vi "VertRead_import_SM1_full_control_100step_camtrigger.vi"() -> ()   [LabVIEW 2021]
uses:
  <vilib>/DAQmx/write.llb/DAQmx Write (Analog 1D DBL NChan 1Samp).vi
  <vilib>/DAQmx/create/channels.llb/DAQmx Create Channel (AO-Voltage-Basic).vi
  <vilib>/Utility/file.llb/Read Delimited Spreadsheet (DBL).vi
  <vilib>/DAQmx/miscellaneous.llb/DAQmx Fill In Error Info.vi
panel:
  in  "Steps_Per_Frame":i32
  out "Raw  Inner Loop Iternation":dbl
  out "Camera":dbl
  out "Trigger_Phase_Iterations":i32
  out "Cam_Trigger_Lo":dbl
  out "Cam_Trigger_Hi":dbl
  out "Sequence Length":i32
  in  "Delay (ADDS 10)":i32
  in  "ICC4C 3 (0-10V)":dbl
  in  "ICC4C 2 (0-10V)":dbl
  in  "ICC4C 1 (0-10V)":dbl
  in  "ICC4C 0 (0-10V)":dbl
  in  "Y2 (-10-10V)":dbl
  in  "X2 (-10-10V)":dbl
  in  "Continue Cycle?":bool
  out "Full Cycles":i32
  out "Mirror_Phase_Iterations":i32
  out "Y1 (-10-10V)":dbl format="%_6g"
  out "X1 (-10-10V)":dbl format="%_6g"
  in  "Blanking (0-10v)":dbl=10.0
  in  "561 (0-10v)":dbl
  in  "514 (0-10v)":dbl
  in  "488 (0-10v)":dbl
  in  "445 (0-10v)":dbl
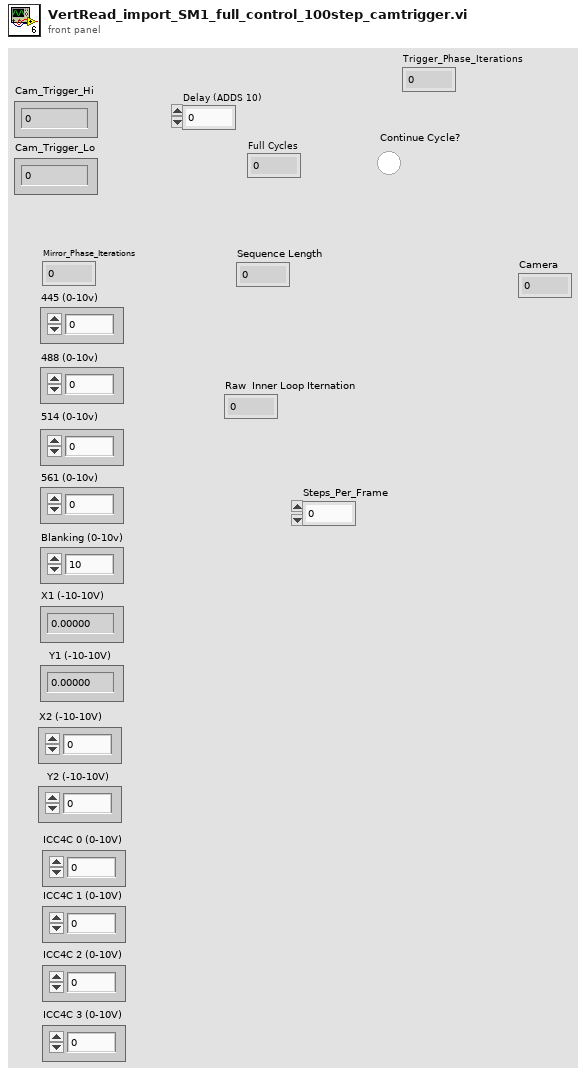
[diagram p1: front panel]
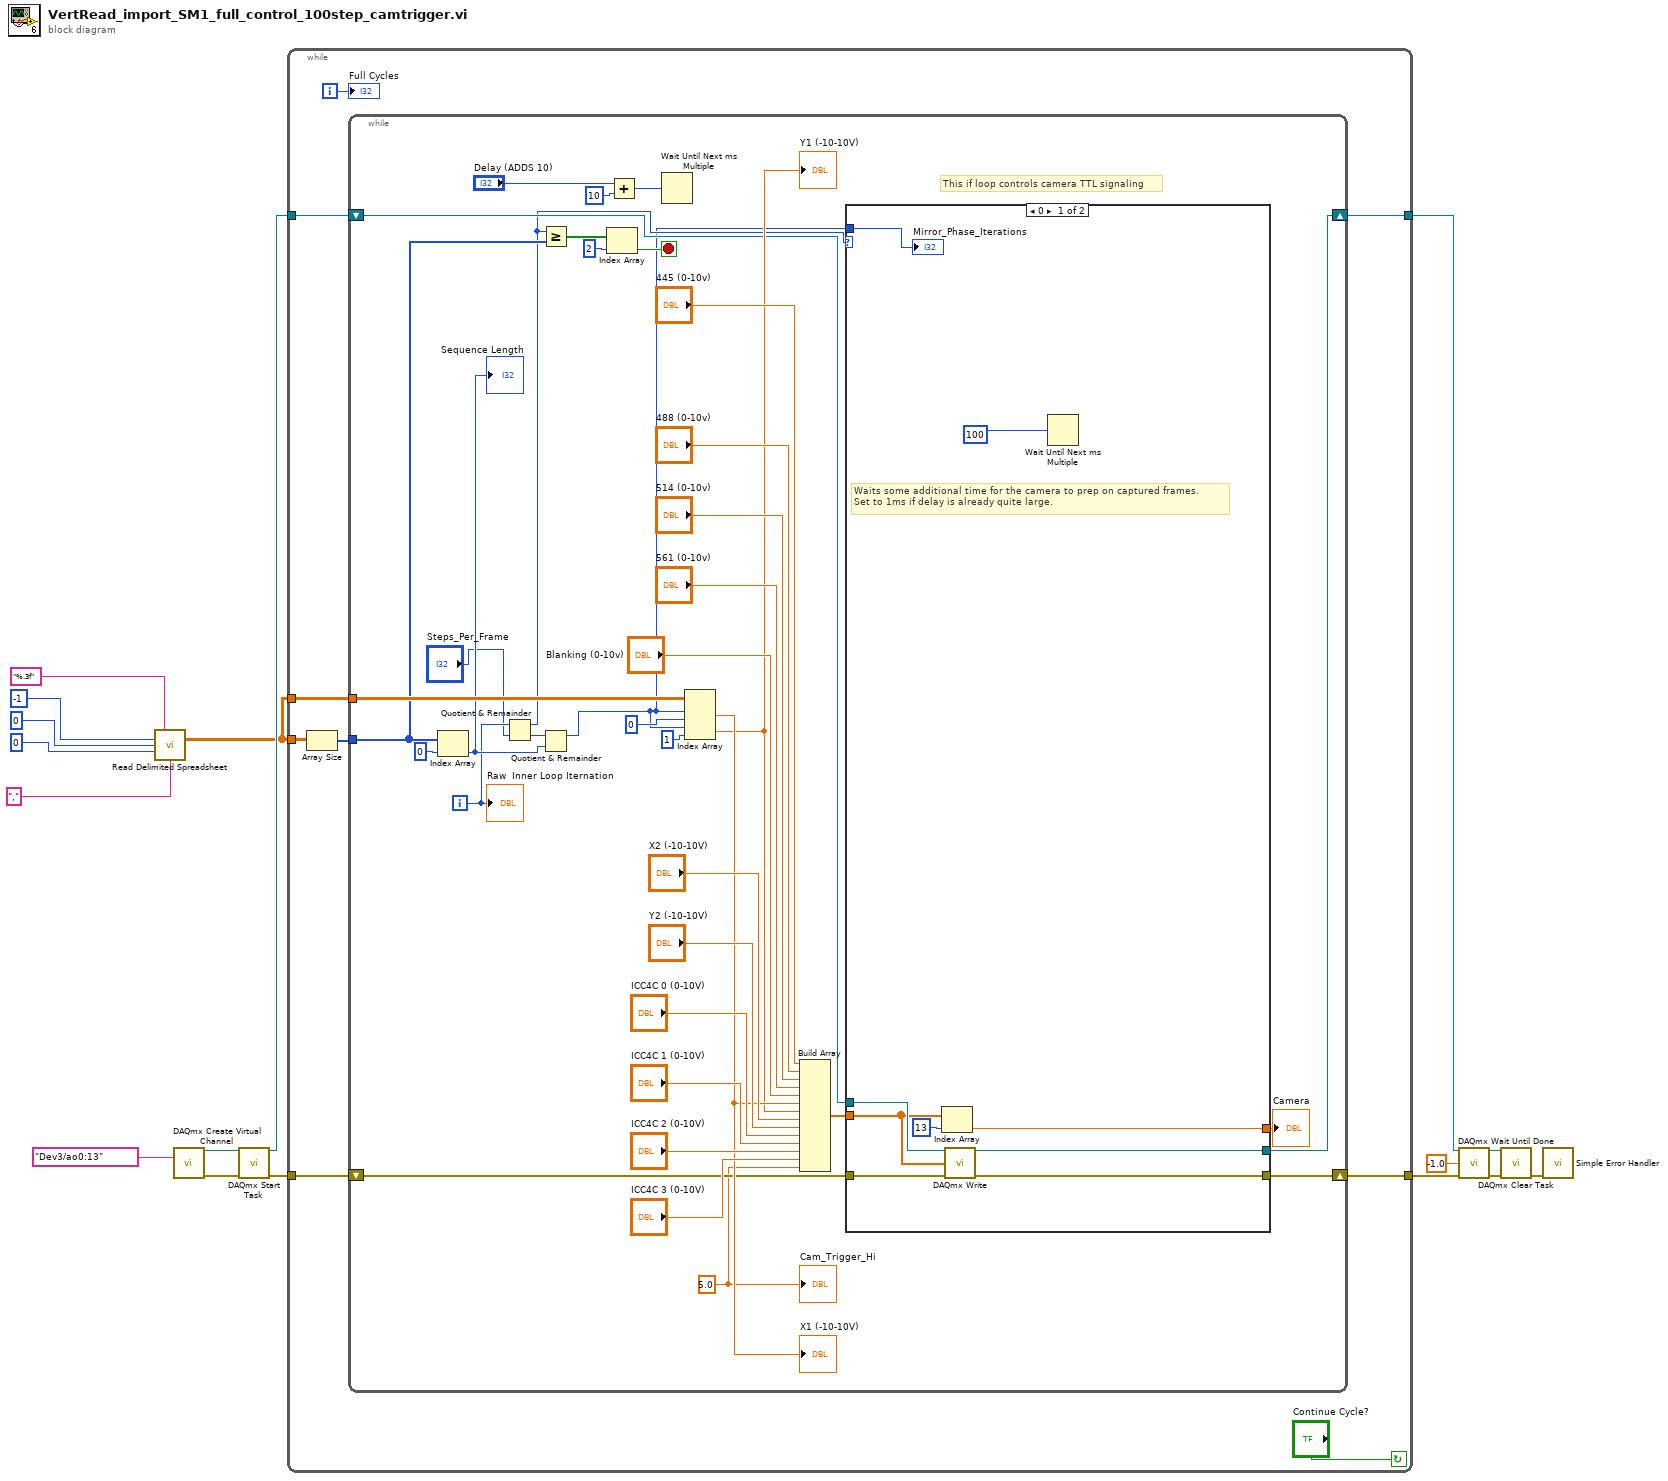
[diagram p0: block diagram]
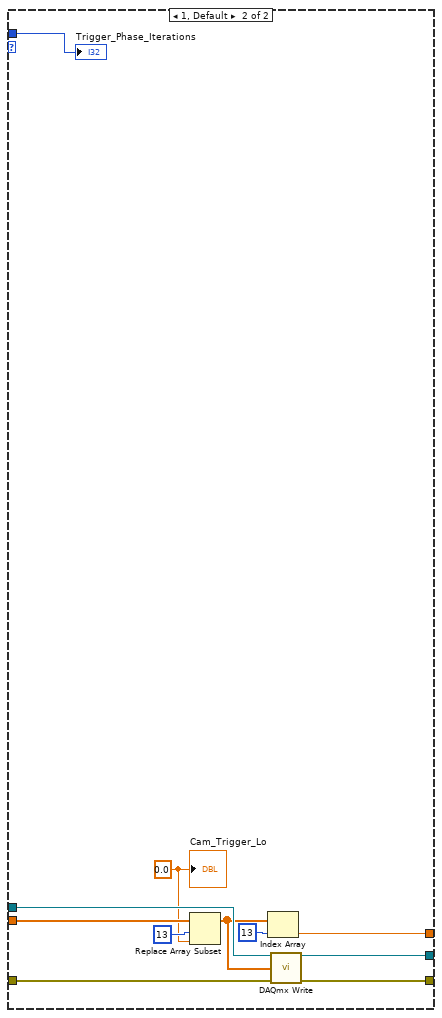
[diagram p2: hidden frame]
diagram:
  n1 = call-poly <vilib>:"Read Delimited Spreadsheet.vi"("format (%.3f)"="%.3f", "number of rows (all:-1)"=-1, "start of read offset (chars.:0)"=0, "max characters/row  (no limit:0)"=0, "delimiter (\\t)"=",") -> ("all rows"=w6:dbl[][])  [unwired: 5 in, 5 out]
  n2 = call-poly <vilib>:"DAQmx Create Virtual Channel.vi"("physical channels"=tag "Dev3/ao0:13") -> ("task out"=w10:refnum<k21>, "error out"=w9:errorcluster)  [unwired: 13 in]
  n3 = call <vilib>:"DAQmx Start Task.vi"("task/channels in"=w10, "error in"=w9) -> ("task out"=w8:refnum<k21>, "error out"=w7:errorcluster)  [unwired: 12 in]
  n4 = while {
    tunnel: [w23] -> w13
    tunnel: [w22] -> w12
    tunnel: w8 -> [w25]
    tunnel: w7 -> [w24]
    tunnel: w6 -> [w20]
    tunnel: w6 -> [w19]
    i -> [w26]
    stop <- "Continue Cycle?" continue-if-true
    n5 = Array Size(array=w20) -> (size(s)=w21:i32[])
    n6 = while {
      shift-right: [w41] -> w23
      shift-left: w25 -> [w40]
      shift-right: [w42] -> w22
      shift-left: w24 -> [w39]
      tunnel: w21 -> [w47]
      tunnel: w19 -> [w49]
      i -> [w36]
      stop <- w50 stop-if-true
      w28 = 5.0
      # "This if loop controls camera TTL signaling"
      n7 = Index Array(array=w47, index=0) -> (element=w45:i32)
      "Sequence Length" <- w45
      n8 = Quotient & Remainder(x=w36, y="Steps_Per_Frame") -> (x-y*floor(x/y)=w37:i32, floor(x/y)=w35:i32)
      n9 = Greater Or Equal?(x=w37, y=w47) -> (x >= y?=w51:bool[])
      n10 = Quotient & Remainder(x=w35, y=w45) -> (x-y*floor(x/y)=w29:i32)  [unwired: 1 out]
      n11 = Index Array(array=w51, index=2) -> (element=w50:bool)
      n12 = Add(x="Delay (ADDS 10)", y=10) -> (x+y=w32:i32)
      n13 = Wait Until Next ms Multiple(millisecond multiple=w32) -> ()  [unwired: 1 out]
      n14 = Index Array(array=w49, index (row) #1=w29, index (col) #1=0, index (row) #2=w29, index (col) #2=1) -> (element #1=w52:dbl, element #2=w48:dbl)
      "X1 (-10-10V)" <- w52
      "Y1 (-10-10V)" <- w48
      n15 = Build Array("445 (0-10v)", "488 (0-10v)", "514 (0-10v)", "561 (0-10v)", "Blanking (0-10v)", w52, w48, "X2 (-10-10V)", "Y2 (-10-10V)", "ICC4C 0 (0-10V)", "ICC4C 1 (0-10V)", "ICC4C 2 (0-10V)", "ICC4C 3 (0-10V)", w28) -> (w43:dbl[])
      n16 = case shown="0" w37 {
        tunnel: w40 -> [w72 w83]
        tunnel: [w69 w82] -> w41
        tunnel: w39 -> [w71 w81]
        tunnel: [w70 w77] -> w42
        tunnel: w43 -> [w68 w80]
        tunnel: w29 -> [w65 w78]
        tunnel: [w66 w74] -> w38
        frame 0 {
          # "Waits some additional time for the camera to prep on captured frames.\nSet to 1ms if delay is already quite large."
          n17 = Index Array(array=w68, index=13) -> (element=w66:dbl)
          n18 = call-poly <vilib>:"DAQmx Write.vi"("task/channels in"=w72, "data"=w68, "error in"=w71) -> ("task out"=w69:refnum<k21>, "error out"=w70:errorcluster)  [unwired: 10 in, 1 out]
          n19 = Wait Until Next ms Multiple(millisecond multiple=100) -> ()  [unwired: 1 out]
          "Mirror_Phase_Iterations" <- w65
        }
        frame 1, Default {
          w73 = 0.0
          n20 = Replace Array Subset(array=w80, new element=w73, index=13) -> (w75:dbl[])
          n21 = Index Array(array=w75, index=13) -> (element=w74:dbl)
          n22 = call-poly <vilib>:"DAQmx Write.vi"("task/channels in"=w83, "data"=w75, "error in"=w81) -> ("task out"=w82:refnum<k21>, "error out"=w77:errorcluster)  [unwired: 10 in, 1 out]
          "Cam_Trigger_Lo" <- w73
          "Trigger_Phase_Iterations" <- w78
        }
      }
      "Camera" <- w38
      "Cam_Trigger_Hi" <- w28
      "Raw  Inner Loop Iternation" <- w36
    }
    "Full Cycles" <- w26
  }
  n23 = call <vilib>:"DAQmx Wait Until Done.vi"("task/channels in"=w13, "timeout (sec)"=-1.0, "error in"=w12) -> ("task out"=w16:refnum<k21>, "error out"=w15:errorcluster)  [unwired: 11 in]
  n24 = call <vilib>:"DAQmx Clear Task.vi"("task in"=w16, "error in"=w15) -> ("error out"=w17:errorcluster)  [unwired: 13 in]
  n25 = call <vilib>:"Simple Error Handler.vi"("error in (no error)"=w17) -> ()  [unwired: 4 in, 5 out]
